vi "KickToBestRobotTactic.vi"(7 "first call":bool, 8 "error in (no error)":errorcluster, 9 "Game in":refnum<class "Game.lvclass">, 10 "Robot":refnum<class "Robot.lvclass">, 11 "KickToBestRobotTactic in":refnum<class "KickToBestRobotTactic.lvclass">) -> (0 "error out":errorcluster, 1 "Game out":refnum<class "Game.lvclass">, 2 "Robot out":refnum<class "Robot.lvclass">, 3 "KickToBestRobotTactic out":refnum<class "KickToBestRobotTactic.lvclass">)   [LabVIEW 2024, in "KickToBestRobotTactic.lvclass"]
uses:
  KickToBestRobotTactic.lvclass
  C:/Users/moise/Documents/GitHub/SSL_AI/Tactic_class/Tactic.lvclass
  Robot_class/Robot.lvclass
  C:/Users/moise/Documents/GitHub/SSL_AI/Object_class/Object.lvclass
  Game_class/Game.lvclass
  Team_class/OffensivePlay.ctl
  KickToPassReceiverTactic_class/KickToPassReceiverTactic.lvclass
  KickTOBestRobotTacticStatesEnum.ctl
  Tactic_class/Tactic.lvclass/Tactic.ctl
  Robot_class/Robot.lvclass/Robot.ctl
  Game_class/Game.lvclass/Game.ctl
  Team_class/Team.lvclass/Team.ctl
  Robot_class/roles.ctl
  Object_class/Object.lvclass/Object.ctl
  Robot_class/tactics.ctl
  Skillbook_class/Skillbook.lvclass/Skillbook.ctl
  Parameters_class/Parameters.lvclass/Parameters.ctl
  Events_class/Events.lvclass/Events.ctl
  Ball_class/Ball.lvclass/Ball.ctl
  KickToBestRobotTactic.lvclass/KickToBestRobotTactic.ctl
  Team_class/Read RobotRef.vi
  Game_class/Read Parameters.lvclass.vi
  Game_class/Read BallRef.vi
  Game_class/Read EventsRef.vi
  Game_class/Read NewParameters.vi
  Events_class/Read kick.vi
  Ball_class/Read velocityNorm.vi
  Parameters_class/Read BallVelToAbortPass.vi
  Object_class/Read position(x,y).vi
  Skillbook_class/Read KickToSkill.vi
  Robot_class/Read kick_x.vi
  Robot_class/Write kick_x.vi
  Game_class/Read Utilities.lvclass.vi
  Game_class/Read OffensiveTeam.vi
  Game_class/Read FieldRef.vi
  Game_class/Read KeeperTeam.vi
  Team_class/Read KeeperPlay.vi
  Team_class/Read OffensivePlay.vi
  Robot_class/Read tactic.vi
  Robot_class/Read id.vi
  Robot_class/Read dest_x.vi
  Robot_class/Read dest_y.vi
  Robot_class/Read dest_orientation.vi
  Robot_class/Read Zone.vi
  Parameters_class/Read AttakingOurselves.vi
  Tactic_class/Read Skillbook.vi
  Write States.vi
  Robot_class/Write tactic.vi
  Robot_class/Write keepDest.vi
  <vilib>/Analysis/_algsub.llb/Vector Norm.vi
  <vilib>/Analysis/_algsub.llb/Real Vector Norm.vi
  Ally_class/Ally.lvclass
  C:/Users/moise/Documents/GitHub/SSL_AI/Team_class/Team.lvclass
  Parameters_class/Parameters.lvclass
  Utilities_class/Utilities.lvclass
  Ball_class/Ball.lvclass
  Field_class/Field.lvclass
  Zone_class/Zone.lvclass
  Skillbook_class/Skillbook.lvclass
  Events_class/Events.lvclass
  KickToSkill_class/KickToSkill.lvclass
  5RobotsSkill_class/5RobotsSkill.lvclass
  ShootTactic_class/ShootTactic.lvclass
panel:
  in  "OneTouchMultiplier":dbl=0.9 format="%#_13g"
  out "x .or. y?":bool
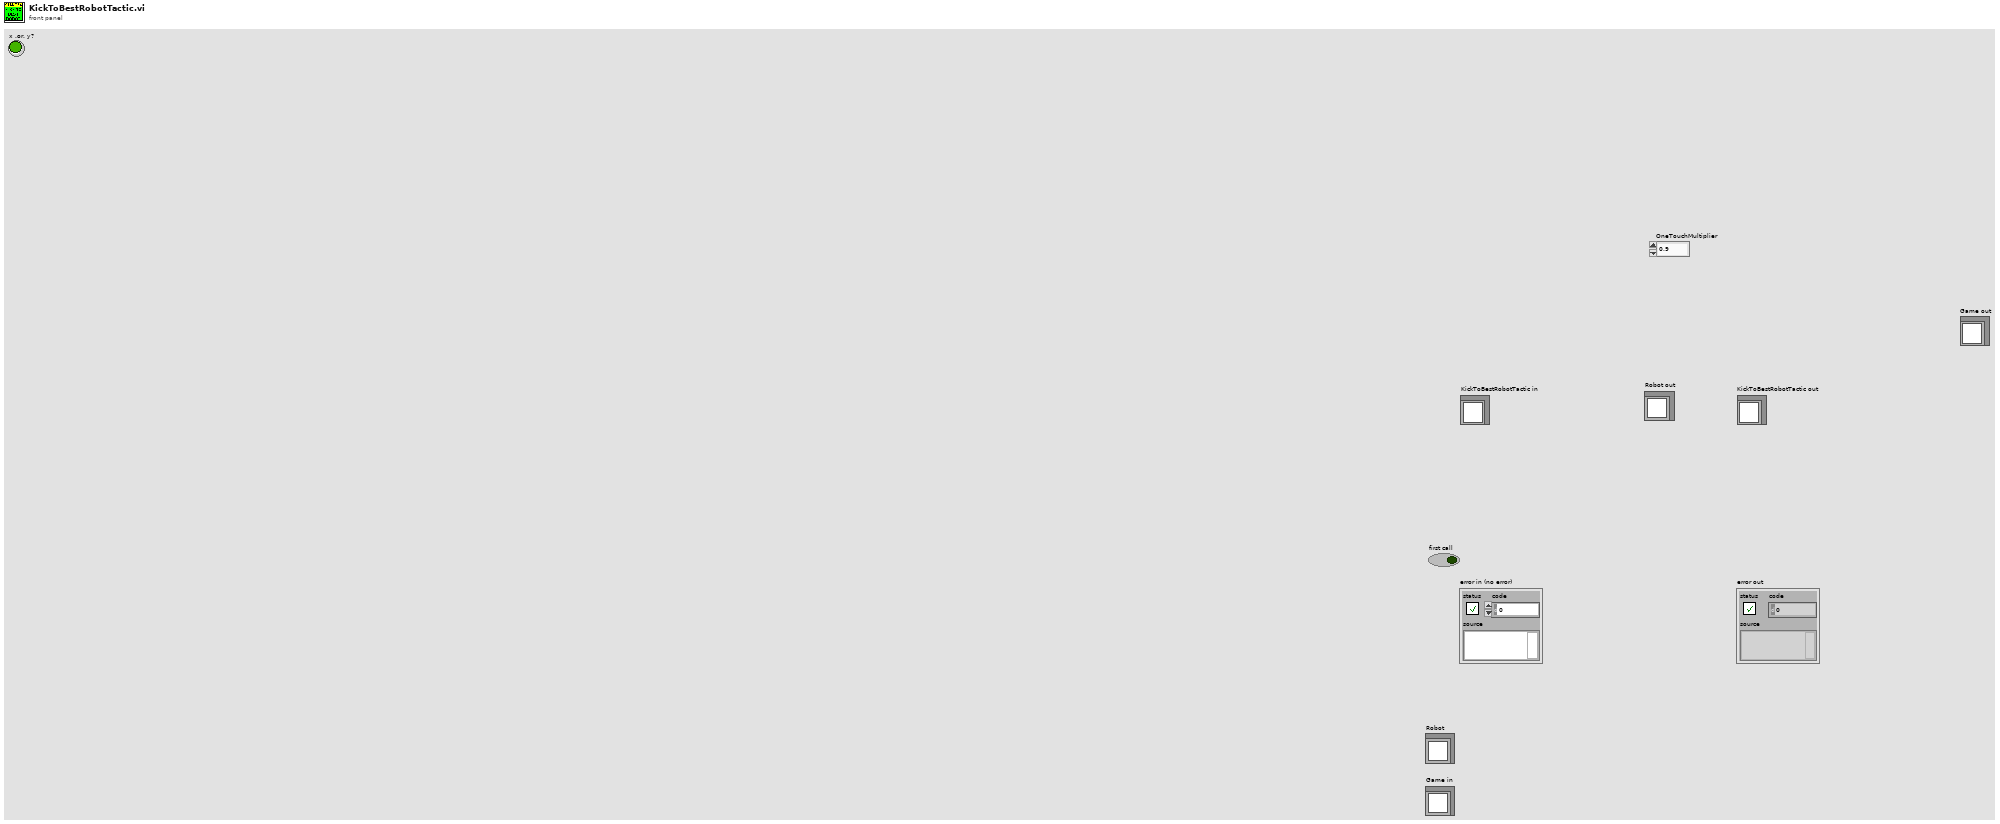
[diagram p1: front panel]
types:
  T1 = typedef "KickToBestRobotTactic.lvclass/KickTOBestRobotTacticStatesEnum.ctl" = enum16{"WaitToPass", "Pass", "Exit"}
  T2 = typedef "OffensivePlay.ctl" = enum16{"5RobotsPassGamePlay", "5PreparePassGame", "5RobotsKeeperGame", "KeeperPassToStriker", "5RobotsNormalGamePlay", "PrepareKeeperPass", "ACBPass", "ABCPass", "PrepareTriplePass", "TableWithStriker", "TableWith2ndStrikerPlay", "PrepareDoublePass", "PrepareRollToPass", "SimplePass", "PreparePass", "PassToStriker", "BallOutOfField", "PassTo2ndStriker", "StopOffensive", "Prepare Penalty Enemy", "EnemyPossessionAtEnemyField", "EnemyPossesionAtOurField", "TestPlay", "PreparePenaltyAlly", "KickPenaltyAlly", "PrepareKickoffAlly", "PrepareKickoffEnemy", "IndirectEnemy", "DirectEnemy", "PreparePassInGame1", "NormalGame", "DirectKick", "Pass", "Halt", "Timeout", "PassPlay", "PenaltyEnemy"}
  T3 = typedef "roles.ctl" = enum16{"SimpleBallPlacement", "BallPlacementAllyPasser", "BallPlacementAllyReceiver", "BallPlacementEnemy", "5Robots5th", "PassBestReceiver", "5Robots4th", "5Robots3rd", "5Robots2nd", "5Robots1st", "PassBestRobot", "WaitPass", "ABCThirdKicker", "ABCFirstKicker", "ABCSecondKicker", "Tabler", "TableFinalizer", "PrepareRollToPassRoller", "PrepareRollToPassReceiver", "SimplePassRoll", "SimplePassRollReceiver", "PenaltyDefense", "PreparePassReceiver 2", "PreparePassReceiver 1", "PassObserver", "Timeout", "Goto", "ZigZag", "None", "BallOutOfField", "DefenderArea", "Duelist", "AttackerStop", "FollowAttacker", "KeeperRole", "KickPenalty", "AttackerAimGoal", "AttackerBlock", "Marker", "Halt", "Shoot", "PassKicker", "PassReceiver", "TestRole", "PenaltyAttacker"}
  T4 = typedef "tactics.ctl" = enum16{"GoToBallPlacementPosition", "PlaceBall", "GoToBallPlacement", "5Robots", "BallPlacementEnemy", "ReceivePassInFuturePoint", "Roller", "PrepareRollToPassRollerGoTo", "PrepareRollToPassReceiverGoTo", "WaitRoll", "PositionToRoll", "PenaltyAttacker", "PassObserver", "PenaltyDefense", "TableReceiverTactic", "Test", "DefendGoal", "Marker", "FollowAttacker", "DefendArea", "Shoot", "AttackerAimGoal", "AttackerBallOutOfField", "AttackerBlock", "AttackerStop", "Duelist", "Halt", "ZigZag", "GoTo", "Timeout", "KickToBestRobot", "KickToPassReceiver", "PositionToReceivePass", "WaitPass", "GoToTarget"}
  T5 = typedef "KeeperPlay.ctl" = enum16{"SimpleBallPlacementAlly", "BallPlacementAlly", "BallPlacementEnemy", "ZigZag", "Goto", "NormalGame", "KeeperPlay", "Halt", "Timeout", "PenaltyEnemy", "TestPlay"}
  T6 = typedef "NewParameters.ctl" = cluster{"PenaltyDistance":dbl, "DistanceAttackerToBackBall":dbl, "Division":enum16{"Div B", "Div A"}, "DistanceToAvoidyEnemyRobot":dbl, "BallPlacementDistance":dbl, "DisatanceBehindBallToStealBall":dbl, "MaxDistanceToPositionKickoff":dbl, "BlockEnemyTarget":bool, "MaxStopVAng":dbl, "DistanceMarkerToEnemy":dbl, "IgnoreDribblerContact":bool, "DistanceToBeginEnemyPosession":dbl, "GoToBallWhenEnemyNotMoving":bool, "EnemyDistanceToReduceVelocity":dbl, "TurnOnEnemyDistanceToReduceVelocity":bool, "EnemyDistanceToShootOutBall":dbl, "DefenseKickBall":bool, "MoreKickToGoal? (0-0.3)":dbl, "ChipKickInEnemyField":bool, "ShootOutRobotId":dbl, "FieldLenghtDenominatorInShootOut":dbl, "AdjustPositionInBallPlacement":bool, "PowerGodPass":dbl, "VelocityAbortEnemyPos":dbl, "MaxDistToBeginPass":dbl, "MinDistToBeginPass":dbl, "VelocityInDirects":dbl, "BadDribblerIDs":i32[], "NewKickToDistanceAroundBall":dbl, "PowerAvoidColisionMarker":dbl, "DistanceToAvoidColisionMarker":dbl, "AvoidBallKick":dbl, "DistanceTryKick":dbl, "SuicideKickDIstance":dbl, "AdjustFirstKickDistance":dbl, "AvoidAimLessKick":dbl, "DistanceToAvoidyEnemyShootRobot ":dbl, "NumberOfMarkers":dbl, "PotField":bool, "PIDLateral":bool, "MinDistanceFirstKickX":dbl, "MinDistanceFirstKickY":dbl, "FractionOfDistToTouchGround\nAfterChipKick":dbl, "FractionOfKickxWhen\nComposedWithKickz":dbl, "Style":T7, "MoveInTurnState":bool, "DistFromEnemyToConsider\nMoveInTurnState":dbl, "CascadePID":bool, "TurnAroundParameters":cluster{"Radius":dbl, "Multiplier":dbl, "ChordAngle":dbl}, "SafeDriveVel":dbl, "DistanceToGoToBackBall":dbl, "minDistanceToNotFinish\nEnemyPossession":dbl, "OneTouchShot":cluster{"angleFactor":dbl, "maxAngle":dbl, "Attack":bool, "Defense":bool}, "OpenAngleToGoal":cluster{"minAngle":dbl, "maxAngle":dbl, "minEvaluation":dbl}, "ShotInterception":cluster{"shotSpeed":dbl, "minEnemySpeed":dbl, "maxEnemySpeed":dbl, "minEvaluation":dbl}, "AllyTeamArray":T8[], "maxDefendersNumber":i32, "Zone":cluster{"GuardPositionArray":dbl[][], "ZoneMidField":dbl[], "CenterForwardWidth":dbl}, "MinEvaluationToShoot":dbl, "PassInterception":cluster{"maxPassSpeed":dbl, "minPassSpeed":dbl, "minEnemySpeed":dbl, "chipPassDistance":dbl, "chipPassEvaluation":dbl, "minEvaluation":dbl, "maxEnemySpeed":dbl}, "PassDistance":cluster{"maxDistance":dbl, "minDistance":dbl}, "receiverSpeed":dbl, "maxBallSpeed":dbl, "slackTime":dbl, "Turning radius":dbl, "Turning v_ang":dbl, "AlignError":cluster{"Distance":dbl, "Orientation":dbl, "V_norm(m/s)":dbl, "V_ang (rad/s)":dbl}, "RobotRadius":dbl, "KickerDistance":dbl, "keeper angle  to cover goalpost":dbl, "a_slide":dbl, "a_roll":dbl, "k_switch":dbl}
  T7 = typedef "Style.ctl" = enum16{"Insanity", "Offensive", "Defensive"}
  T8 = typedef "AllyTeam.ctl" = enum16{"Keeper", "Defender", "Attacker"}
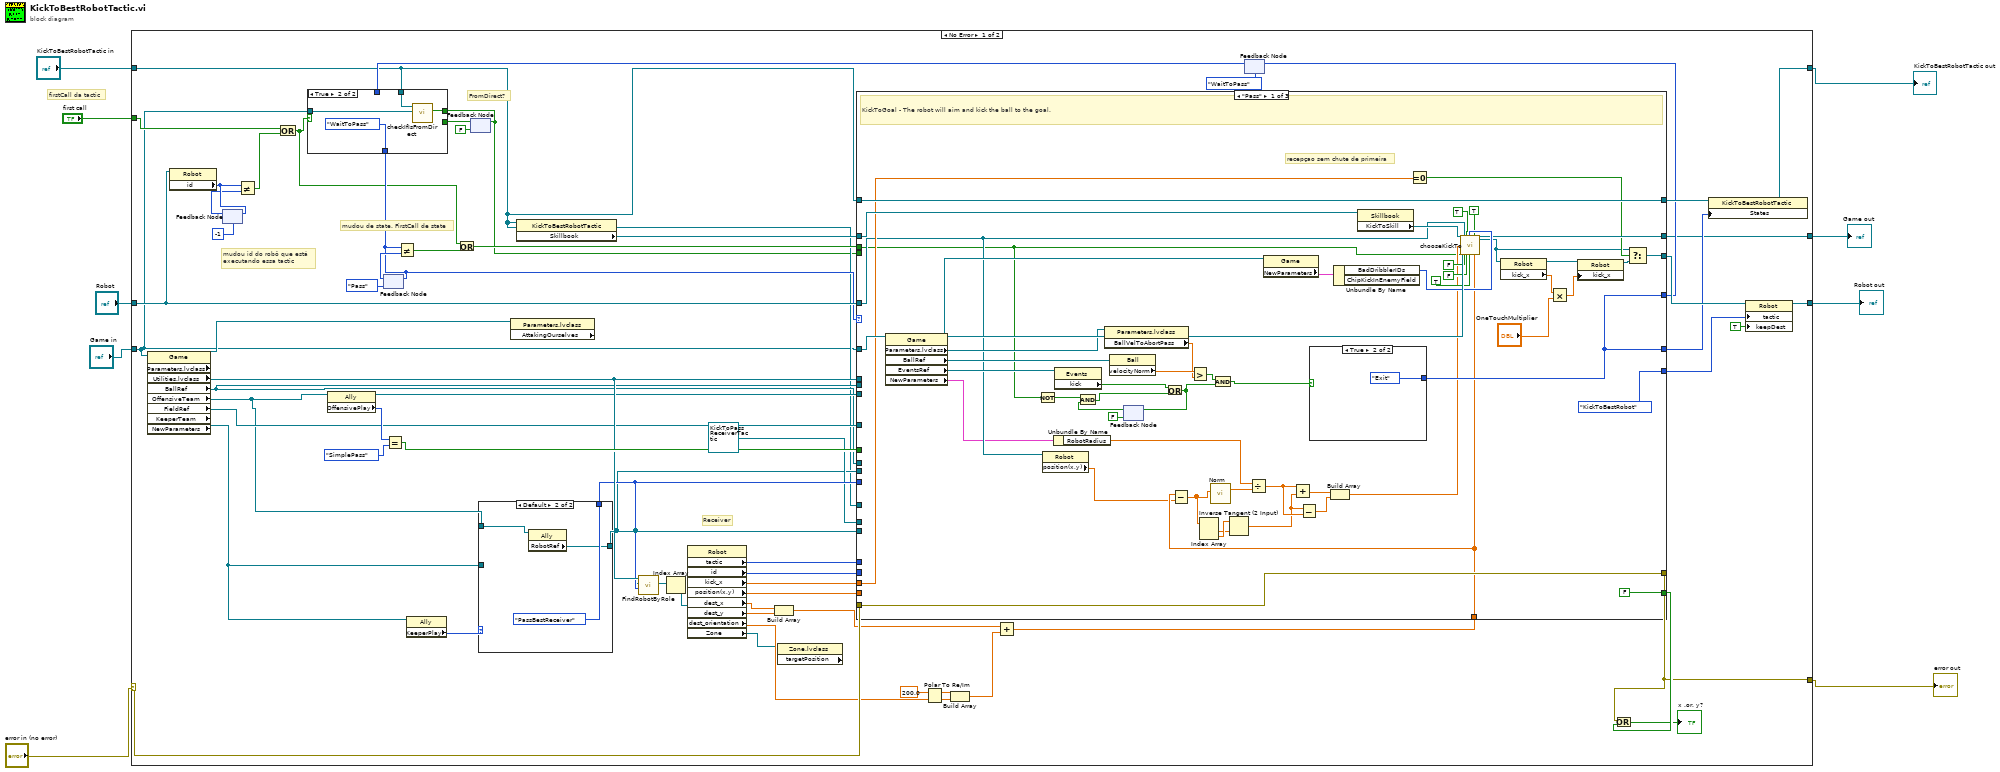
[diagram p0: block diagram]
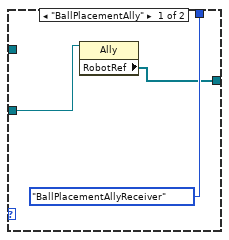
[diagram p2: hidden frame]
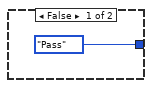
[diagram p4: hidden frame]
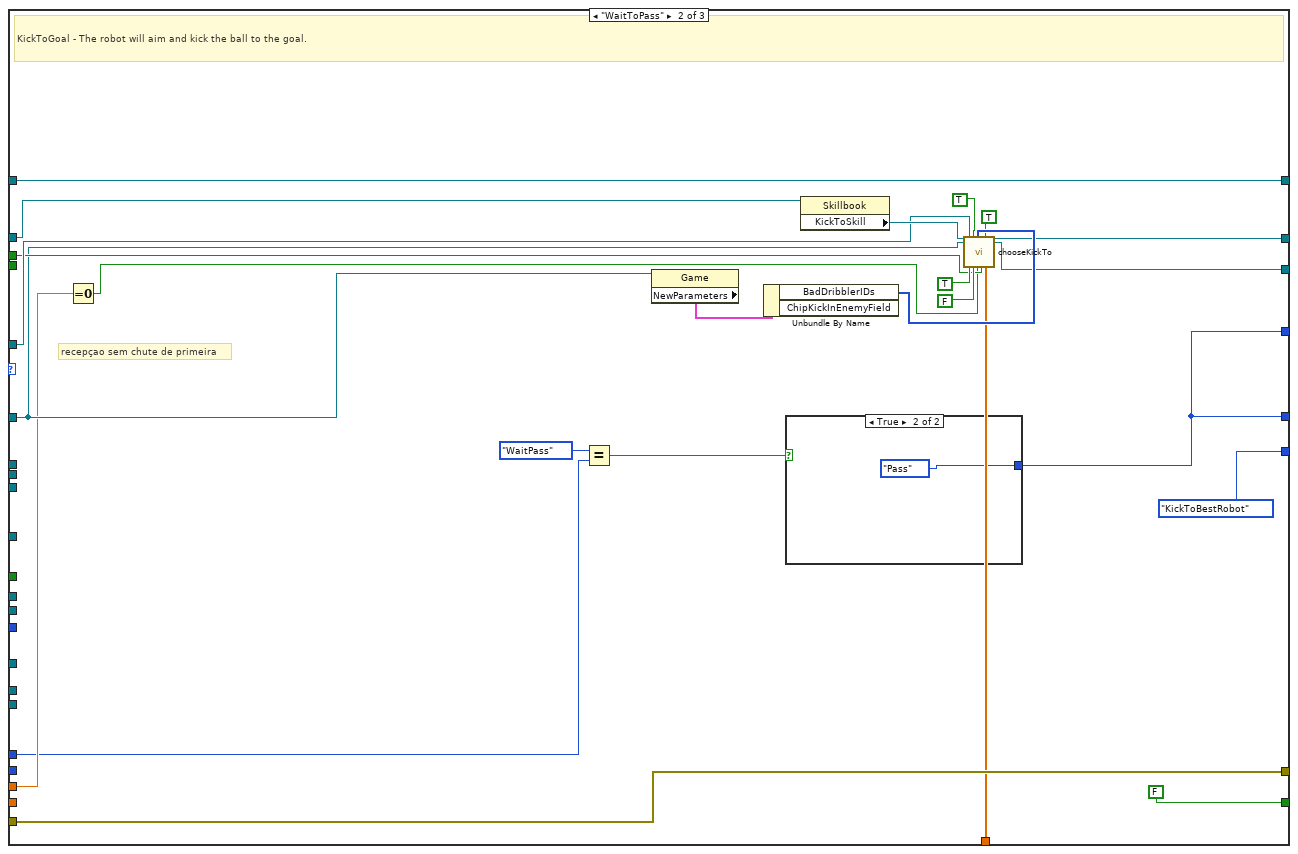
[diagram p5: hidden frame]
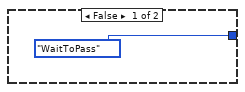
[diagram p6: hidden frame]
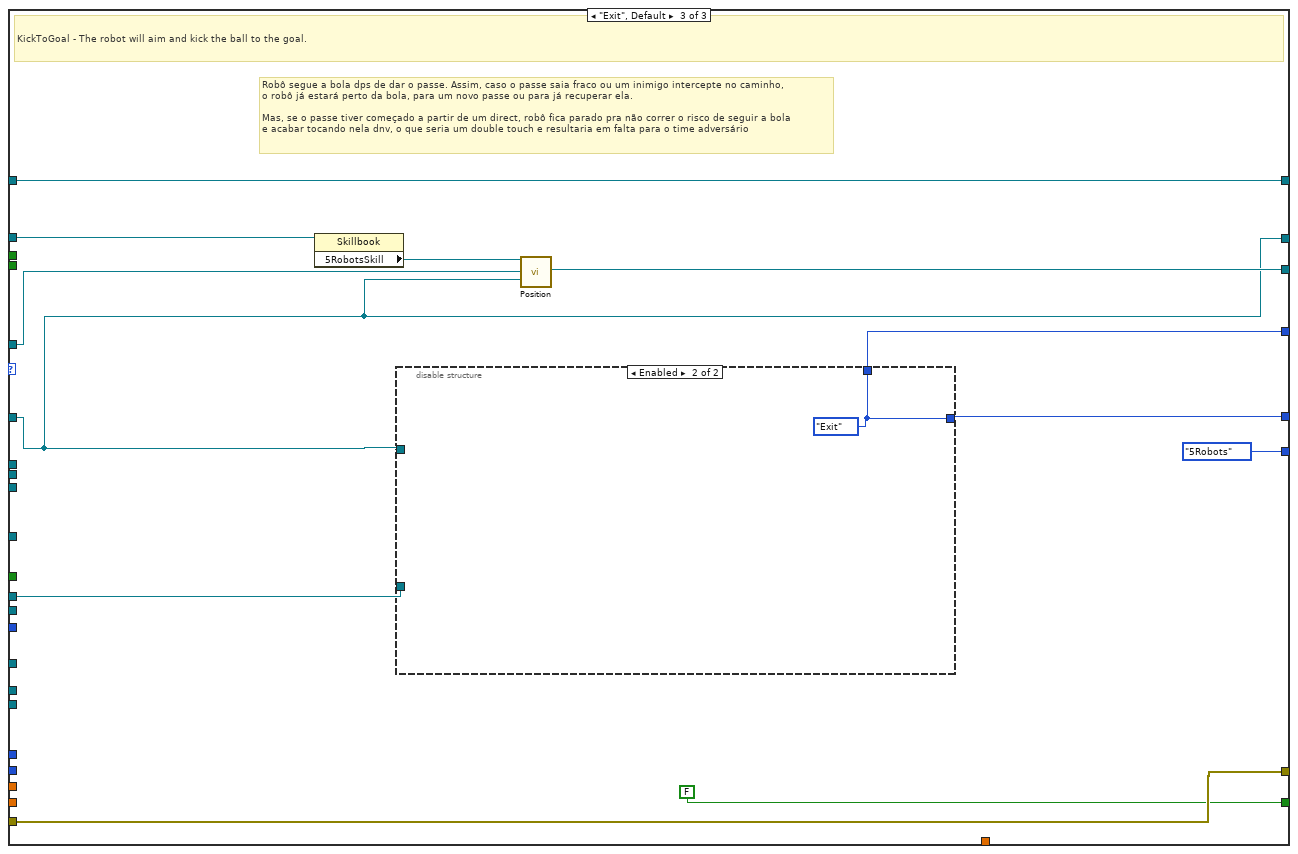
[diagram p7: hidden frame]
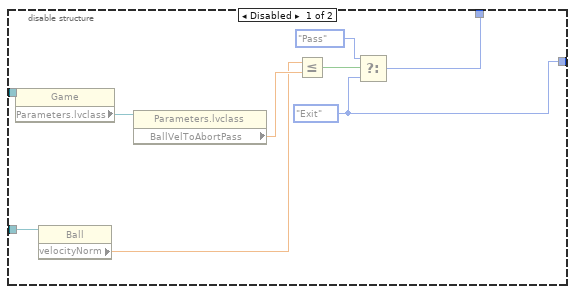
[diagram p8: hidden frame]
diagram:
  # "firstCall da tactic"
  n1 = case shown="No Error" "error in (no error)" {
    selector: "error in (no error)" -> [w66 w191]
    tunnel: [w67 w191] -> w6
    tunnel: [w68 w190] -> w8
    tunnel: "KickToBestRobotTactic in" -> [w27 w190]
    tunnel: "Robot" -> [w46 w189]
    tunnel: "Game in" -> [w26 _]
    tunnel: [w63 w189] -> w7
    tunnel: "first call" -> [w42 _]
    tunnel: [w39 _] -> w1
    frame No Error {
      # "FromDirect?"
      # "mudou de state. FirstCall de state"
      # "mudou id do robô que está\nexecutando essa tactic"
      # "Receiver"
      n2 = property class="Game" props=["Parameters.lvclass", "Utilities.lvclass", "BallRef", "OffensiveTeam", "FieldRef", "KeeperTeam", "NewParameters"](reference=w26) -> ("Parameters.lvclass"=w57:refnum<class "Parameters.lvclass">, "Utilities.lvclass"=w60:refnum<class "Utilities.lvclass">, "BallRef"=w40:refnum<class "Ball.lvclass">, "OffensiveTeam"=w37:refnum<class "Ally.lvclass">, "FieldRef"=w55:refnum<class "Field.lvclass">, "KeeperTeam"=w36:refnum<class "Ally.lvclass">)  [unwired: 1 in, 3 out]
      n3 = property class="Robot"(reference=w46) -> ("id"=w45:i32)  [unwired: 1 in, 2 out]
      n4 = feedback-in #1(w45) -> ()
      n5 = feedback #1(-1 ("id")) -> (w44:i32)
      n6 = Not Equal?(x=w45, y=w44) -> (x != y?=w41:bool)
      n7 = Compound Arithmetic op=OR(w42, w41) -> (w30:bool)
      n8 = property class="Ally"(reference=w37) -> (reference out=w56:refnum<class "Ally.lvclass">, "OffensivePlay"=w59:T2)  [unwired: 1 in, 1 out]
      n9 = feedback #2(KickTOBestRobotTacticStatesEnum."Pass" ("States")) -> (w33:T1)
      n10 = Equal?(x=w59, y=OffensivePlay."SimplePass" ("OffensivePlay")) -> (x = y?=w61:bool)
      n11 = property class="Ally"(reference=w36) -> ("KeeperPlay"=w38:T5)  [unwired: 1 in, 2 out]
      n12 = feedback #3(FALSE ("FromPreparePass")) -> (w25:bool)
      n13 = case shown="Default" w38 {
        tunnel: [roles."BallPlacementAllyReceiver" ("role") roles."PassBestReceiver" ("role")] -> w54
        tunnel: [w74 w77] -> w35
        tunnel: w37 -> [_ w76]
        tunnel: w36 -> [w73 _]
        frame "BallPlacementAlly" {
          n14 = property class="Ally"(reference=w73) -> ("RobotRef"=w74:refnum<class "Robot.lvclass">[])  [unwired: 1 in, 2 out]
        }
        frame Default {
          n15 = property class="Ally"(reference=w76) -> ("RobotRef"=w77:refnum<class "Robot.lvclass">[])  [unwired: 1 in, 2 out]
        }
      }
      n16 = property class="Parameters.lvclass" props=["AttakingOurselves"](reference=w57) -> ()  [unwired: 1 in, 3 out]
      n17 = property class="KickToBestRobotTactic"(reference=w27) -> ("Skillbook"=w70:refnum<class "Skillbook.lvclass">)  [unwired: 1 in, 2 out]
      n18 = call "FindRobotByRole.vi"("role"=w54, "RobotRef"=w35, "Utilities in"=w60) -> ("Robots"=w52:refnum<class "Robot.lvclass">[])  [unwired: 5 in, 3 out]
      n19 = Index Array(array=w52) -> (element=w50:refnum<class "Robot.lvclass">)  [unwired: 1 in]
      n20 = property class="Robot"(reference=w50) -> ("tactic"=w15:T4, "id"=w16:i32, "kick_x"=w22:dbl, "position(x,y)"=w34:dbl[], "dest_x"=w18:dbl, "dest_y"=w17:dbl, "dest_orientation"=w19:dbl, "Zone"=w14:refnum<class "Zone.lvclass">)  [unwired: 1 in, 2 out]
      n21 = Build Array(w18, w17) -> (w13:dbl[])
      n22 = property class="Zone.lvclass" props=["targetPosition"](reference=w14) -> ()  [unwired: 1 in, 3 out]
      n23 = Polar To Re/Im(2:w19, 3:200.0 ("r")) -> (0:w20:dbl, 1:w21:dbl)
      n24 = Build Array(w21, w20) -> (w51:dbl[])
      n25 = Add(x=w13, y=w51) -> (x+y=w58:dbl[])
      n26 = feedback #4(KickTOBestRobotTacticStatesEnum."WaitToPass" ("States")) -> (w65:T1)
      n27 = case shown="True" w30 {
        tunnel: [w80 KickTOBestRobotTacticStatesEnum."WaitToPass" ("States")] -> w32
        tunnel: w65 -> [w80 _]
        tunnel: w27 -> [_ w83]
        tunnel: w26 -> [_ w82]
        tunnel: [w79 w81] -> w23
        tunnel: w25 -> [w79 _]
        frame False {
        }
        frame True {
          n28 = call "checkIfIsFromDirect.vi"("Game"=w82, "KickToBestRobotTactic in"=w83) -> ("FromPreparePass"=w81:bool)  [unwired: 7 in, 2 out]
        }
      }
      n29 = feedback-in #2(w32) -> ()
      n30 = Not Equal?(x=w32, y=w33) -> (x != y?=w28:bool)
      n31 = Or(x=w30, y=w28) -> (x .or. y?=w29:bool)
      n32 = feedback-in #3(w23) -> ()
      n33 = case shown="\"Pass\"" w32 {
        tunnel: [FALSE ("Stop Loop?") FALSE ("Stop Loop?") FALSE ("Stop Loop?")] -> w72
        tunnel: w66 -> [w137 w163 w176]
        tunnel: [w137 w163 w176] -> w67
        tunnel: w70 -> [w136 w162 w178]
        tunnel: w46 -> [w105 w150 w170]
        tunnel: [w115 w153 w171] -> w64
        tunnel: [w135 w161 w177] -> w69
        tunnel: w27 -> [w135 w161 w177]
        tunnel: w26 -> [w123 w148 w168]
        tunnel: [w133 w160 w174] -> w48
        tunnel: w40 -> [_ _ w169]
        tunnel: w60 -> [_ _ _]
        tunnel: w61 -> [_ _ _]
        tunnel: w58 -> [w104 w147 _]
        tunnel: w56 -> [_ _ _]
        tunnel: w55 -> [_ _ _]
        tunnel: w54 -> [_ _ _]
        tunnel: w35 -> [_ _ _]
        tunnel: w27 -> [_ _ _]
        tunnel: refnum<class "KickToPassReceiverTactic.lvclass"> refnum ("KickToPassReceiverTactic in") -> [_ _ _]
        tunnel: [w133 w160 w173] -> w47
        tunnel: w40 -> [_ _ _]
        tunnel: [w125 w152 w168] -> w39
        tunnel: w35 -> [_ _ _]
        tunnel: w34 -> [_ _ _]
        tunnel: w29 -> [w87 w149 _]
        tunnel: w23 -> [_ _ _]
        tunnel: w22 -> [w122 w146 _]
        tunnel: w16 -> [_ _ _]
        tunnel: w15 -> [_ w144 _]
        tunnel: [tactics."KickToBestRobot" ("tactic") tactics."KickToBestRobot" ("tactic") tactics."5Robots" ("tactic")] -> w12
        frame "Pass" {
          # "recepçao sem chute de primeira"
          # "KickToGoal - The robot will aim and kick the ball to the goal."
          n34 = property class="Game"(reference=w123) -> (reference out=w131:refnum<class "Game.lvclass">, "Parameters.lvclass"=w117:refnum<class "Parameters.lvclass">, "BallRef"=w120:refnum<class "Ball.lvclass">, "EventsRef"=w134:refnum<class "Events.lvclass">, "NewParameters"=w102:T6)  [unwired: 1 in, 1 out]
          n35 = Not(x=w87) -> (.not. x?=w88:bool)
          n36 = property class="Robot"(reference=w105) -> ("position(x,y)"=w103:dbl[])  [unwired: 1 in, 2 out]
          n37 = Unbundle By Name(w102) -> ("RobotRadius"=w101:dbl)
          n38 = property class="Events"(reference=w134) -> ("kick"=w91:bool)  [unwired: 1 in, 2 out]
          n39 = property class="Parameters.lvclass"(reference=w117) -> ("BallVelToAbortPass"=w116:dbl)  [unwired: 1 in, 2 out]
          n40 = property class="Ball"(reference=w120) -> ("velocityNorm"=w118:dbl)  [unwired: 1 in, 2 out]
          n41 = feedback #5(FALSE) -> (w86:bool)
          n42 = And(x=w88, y=w86) -> (x .and. y?=w85:bool)
          n43 = Or(x=w91, y=w85) -> (x .or. y?=w90:bool)
          n44 = feedback-in #5(w90) -> ()
          n45 = Subtract(x=w104, y=w103) -> (x-y=w98:dbl[])
          n46 = Greater?(x=w118, y=w116) -> (0:w119:bool)
          n47 = Index Array(array=w98) -> (element #1=w96:dbl, element #2=w97:dbl)  [unwired: 2 in]
          n48 = call "Norm.vi"("2D vector"=w98) -> ("Modulo"=w100:dbl)  [unwired: 8 in, 2 out]
          n49 = And(x=w119, y=w90) -> (x .and. y?=w121:bool)
          n50 = Inverse Tangent (2 Input)(1:w96, 2:w97) -> (0:w95:dbl)
          n51 = Divide(x=w101, y=w100) -> (x/y=w99:dbl)
          n52 = property class="Game"(reference=w131) -> ("NewParameters"=w130:T6)  [unwired: 1 in, 2 out]
          n53 = Add(x=w99, y=w95) -> (x+y=w94:dbl)
          n54 = Subtract(x=w95, y=w99) -> (x-y=w93:dbl)
          n55 = case shown="True" w121 {
            tunnel: [KickTOBestRobotTacticStatesEnum."Pass" ("States") KickTOBestRobotTacticStatesEnum."Exit" ("States")] -> w133
            frame False {
            }
            frame True {
            }
          }
          n56 = Build Array(w94, w93) -> (w92:dbl[])
          n57 = Unbundle By Name(w130) -> ("BadDribblerIDs"=w129:i32[])  [unwired: 1 out]
          n58 = property class="Skillbook"(reference=w136) -> ("KickToSkill"=w132:refnum<class "KickToSkill.lvclass">)  [unwired: 1 in, 2 out]
          n59 = Equal To 0?(x=w122) -> (x = 0?=w112:bool)
          n60 = call "chooseKickTo.vi"("KickToSkill in"=w132, "Game in"=w131, "target gap"=w92, "Robot"=w105, "KickForce 0?"=FALSE, "use criteria?"=TRUE, "ForceInGame"=FALSE, "BadDribblerIDs"=w129, "pass?"=TRUE ("ForceInGame"), "firstCall"=w87, "ChipKickInEnemyField"=TRUE, "Target"=w104) -> ("Game out"=w125:refnum<class "Game.lvclass">, "Robot out"=w111:refnum<class "Robot.lvclass">)  [unwired: 14 in]
          n61 = property class="Robot"(reference=w111) -> (reference out=w110:refnum<class "Robot.lvclass">, "kick_x"=w109:dbl)  [unwired: 1 in, 1 out]
          n62 = Multiply(x=w109, y="OneTouchMultiplier") -> (x*y=w108:dbl)
          n63 = property class="Robot"(reference=w110, "kick_x"=w108) -> (reference out=w114:refnum<class "Robot.lvclass">)  [unwired: 1 in, 1 out]
          n64 = Select(t=w111, s=w112, f=w114) -> (s? t:f=w115:refnum<class "Robot.lvclass">)
        }
        frame "WaitToPass" {
          # "recepçao sem chute de primeira"
          # "KickToGoal - The robot will aim and kick the ball to the goal."
          n65 = Equal To 0?(x=w146) -> (x = 0?=w145:bool)
          n66 = Equal?(x=tactics."WaitPass", y=w144) -> (x = y?=w142:bool)
          n67 = property class="Game"(reference=w148) -> ("NewParameters"=w158:T6)  [unwired: 1 in, 2 out]
          n68 = Unbundle By Name(w158) -> ("BadDribblerIDs"=w157:i32[])  [unwired: 1 out]
          n69 = case shown="True" w142 {
            tunnel: [KickTOBestRobotTacticStatesEnum."WaitToPass" ("States") KickTOBestRobotTacticStatesEnum."Pass" ("States")] -> w160
            frame False {
            }
            frame True {
            }
          }
          n70 = property class="Skillbook"(reference=w162) -> ("KickToSkill"=w159:refnum<class "KickToSkill.lvclass">)  [unwired: 1 in, 2 out]
          n71 = call "chooseKickTo.vi"("KickToSkill in"=w159, "Game in"=w148, "Robot"=w150, "KickForce 0?"=TRUE, "use criteria?"=TRUE, "ForceInGame"=FALSE, "BadDribblerIDs"=w157, "pass?"=w145, "firstCall"=w149, "ChipKickInEnemyField"=TRUE, "Target"=w147) -> ("Game out"=w152:refnum<class "Game.lvclass">, "Robot out"=w153:refnum<class "Robot.lvclass">)  [unwired: 15 in]
        }
        frame "Exit", Default {
          # "Robô segue a bola dps de dar o passe. Assim, caso o passe saia fraco ou um inimigo intercepte no caminho,\no robô já estará perto da bola, para um novo passe ou para já recuperar ela.\n\nMas, se o passe tiver começado a partir de um direct, robô fica parado pra não correr o risco de seguir a bola\ne acabar tocando nela dnv, o que seria um double touch e resultaria em falta para o time adversário"
          # "KickToGoal - The robot will aim and kick the ball to the goal."
          n72 = property class="Skillbook"(reference=w178) -> ("5RobotsSkill"=w172:refnum<class "5RobotsSkill.lvclass">)  [unwired: 1 in, 2 out]
          n73 = disable-structure shown="Enabled" {
            disable-tunnel: w169 -> [w187 _]
            disable-tunnel: [w185 w188] -> w174
            disable-tunnel: [w183 w188] -> w173
            disable-tunnel: w168 -> [w182 _]
            frame Disabled {
              w185 = KickTOBestRobotTacticStatesEnum."Exit" ("States")
              n74 = property class="Game"(reference=w182) -> ("Parameters.lvclass"=w181:refnum<class "Parameters.lvclass">)  [unwired: 1 in, 2 out]
              n75 = property class="Ball"(reference=w187) -> ("velocityNorm"=w179:dbl)  [unwired: 1 in, 2 out]
              n76 = property class="Parameters.lvclass"(reference=w181) -> ("BallVelToAbortPass"=w180:dbl)  [unwired: 1 in, 2 out]
              n77 = Less Or Equal?(x=w179, y=w180) -> (x <= y?=w186:bool)
              n78 = Select(t=KickTOBestRobotTacticStatesEnum."Pass" ("States"), s=w186, f=w185) -> (s? t:f=w183:T1)
            }
            frame Enabled {
              w188 = KickTOBestRobotTacticStatesEnum."Exit" ("States")
            }
          }
          n79 = call-dynamic "Position.vi"("object in"=w172, "Robot"=w170, "Game"=w168) -> ("Robot out"=w171:refnum<class "Robot.lvclass">)  [unwired: 14 in, 2 out]
        }
      }
      n80 = feedback-in #4(w47) -> ()
      n81 = Or(x=w67, y=w72) -> (x .or. y?=→"x .or. y?":bool)
      n82 = property class="KickToBestRobotTactic"(reference=w69, "States"=w48) -> (reference out=w68:refnum<class "KickToBestRobotTactic.lvclass">)  [unwired: 1 in, 1 out]
      n83 = property class="Robot"(reference=w64, "tactic"=w12, "keepDest"=TRUE) -> (reference out=w63:refnum<class "Robot.lvclass">)  [unwired: 1 in, 1 out]
    }
    frame Error {
    }
  }
  "error out" <- w6
  "KickToBestRobotTactic out" <- w8
  "Robot out" <- w7
  "Game out" <- w1
